vi "DISP_ANN_FREQ_STAT.vi"(0 "VISA IN":refnum<visa-resource-name>, 5 "error in":errorcluster, 7 "On|Off":bool) -> (14 "VISA Out":refnum<visa-resource-name>, 19 "error out":errorcluster)   [LabVIEW 2018, in "PNA-X.lvlib"]
doc: "DISPlay:ANNotation:FREQuency[:STATe] <ON | OFF> \n(Read-Write) Turns frequency information on the display title bar ON or OFF for all windows. \nParameters \n<ON | OFF> ON (or 1) - turns frequency annotation ON. \nOFF (or 0) - turns frequency annotation OFF. \nExamples DISP:ANN:FREQ ON \ndisplay:annotation:frequency:state off \nQuery Syntax DISPlay:ANNotation:FREQuency[:STATe]? \nReturn Type Boolean (1 = ON, 0 = OFF) \nDefault ON (1)"
uses:
  PNA-X.lvlib
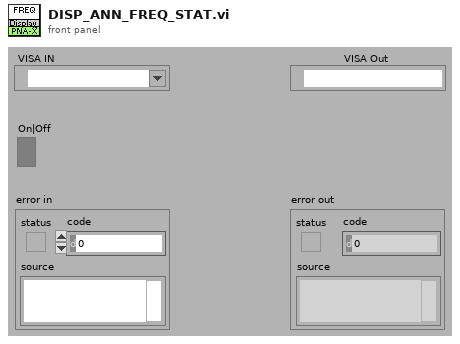
[diagram p1: front panel]
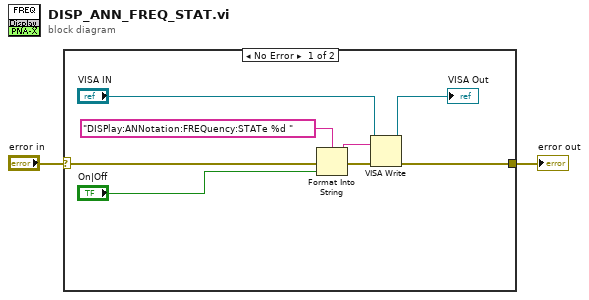
[diagram p0: block diagram]
diagram:
  n1 = case shown="No Error" "error in" {
    selector: "error in" -> [w10 w11]
    tunnel: [w5 w11] -> w1
    frame No Error {
      n2 = Format Into String(format string="DISPlay:ANNotation:FREQuency:STATe %d " ("Cmdline"), error in=w10, "On|Off") -> (resulting string=w8:string, error out=w9:errorcluster)  [unwired: 1 in]
      n3 = VISA Write(VISA resource name="VISA IN", write buffer=w8, error in (no error)=w9) -> (VISA resource name out=→"VISA Out":refnum<visa-resource-name>, error out=w5:errorcluster)  [unwired: 1 out]
    }
    frame Error {
    }
  }
  "error out" <- w1
